vi "CreateMessage.vi"(8 "Calculate Checksum":bool, 9 "array":u8[](array[numeric]), 10 "Command":u8 format="%x") -> (2 "Message":u8[](array[numeric]) format="%x")   [LabVIEW 2014]
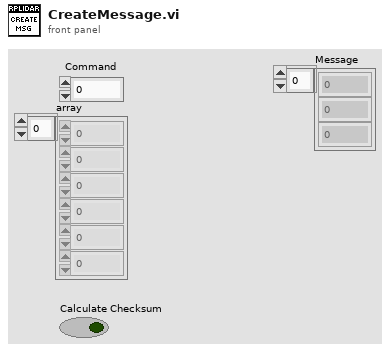
[diagram p1: front panel]
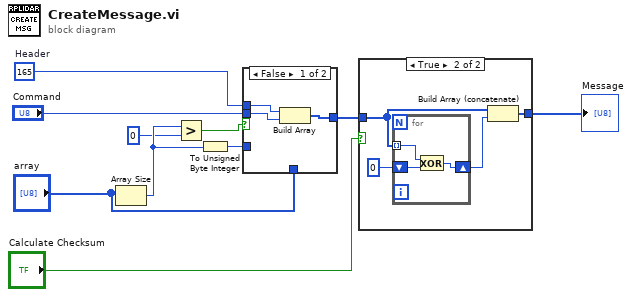
[diagram p0: block diagram]
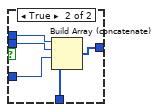
[diagram p3: hidden frame]
diagram:
  w10 = u8 165  # Header
  n1 = Array Size(array="array") -> (size(s)=w4:i32)
  n2 = Greater?(x=w4, y=0) -> (0:w5:bool)
  n3 = To Unsigned Byte Integer(number=w4) -> (unsigned 8bit integer=w6:u8)
  n4 = case shown="False" w5 {
    tunnel: w10 -> [w12 w18]
    tunnel: [w13 w17] -> w8
    tunnel: "Command" -> [w11 w16]
    tunnel: "array" -> [_ w15]
    tunnel: w6 -> [_ w14]
    frame False {
      n5 = Build Array(w12, w11) -> (w13:u8[])
    }
    frame True {
      n6 = Build Array (concatenate)(w18, w16, w14, w15) -> (w17:u8[])
    }
  }
  n7 = case shown="True" "Calculate Checksum" {
    tunnel: [w19 w23] -> w9
    tunnel: w8 -> [w19 w21]
    frame False {
    }
    frame True {
      n8 = for {
        shift-right: [w26] -> w20
        shift-left: u8 0 -> [w25]
        tunnel: w21 -> [w24] mode=indexing
        n9 = Exclusive Or(1:w25, 2:w24) -> (0:w26:u8)
      }
      n10 = Build Array (concatenate)(w21, w20) -> (w23:u8[])
    }
  }
  "Message" <- w9
